vi "Identify Action.vi"(8 "error in (no error)":errorcluster, 10 "Item Tag":string) -> (0 "error out":errorcluster, 3 "RCM_Actions out":refnum<class "RCM_Actions.lvclass">)   [LabVIEW 2016, in "Assert API Components.lvlib" / "Assert Display.lvlib" / "Main Display.lvlib" / "RCM_Actions.lvclass"]
uses:
  RCM_Actions.lvclass
  Change Column Header/Change Column Header.lvclass
  D:/Work/Projects/actor_assert_api/Main Display/Right Click Menu Actions/RCM_Actions.lvclass
  Change Column Header/Change Column Header.lvclass/Change Column Header.ctl
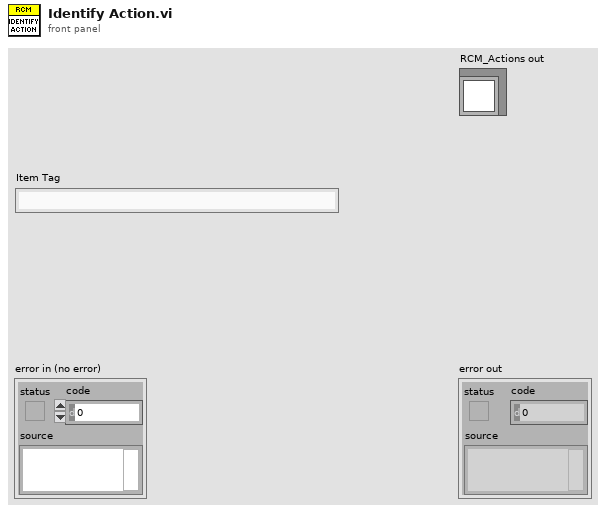
[diagram p1: front panel]
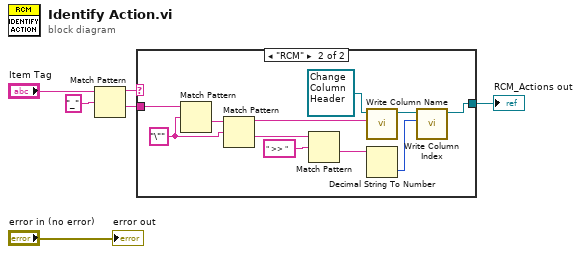
[diagram p0: block diagram]
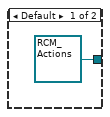
[diagram p2: hidden frame]
diagram:
  n1 = Match Pattern(string="Item Tag", regular expression="_") -> (before substring=w3:string, after substring=w4:string)  [unwired: 1 in, 2 out]
  n2 = case shown="\"RCM\"" w3 {
    tunnel: w4 -> [_ w13]
    tunnel: [refnum<class "RCM_Actions.lvclass"> refnum ("RCM_Actions out") w10] -> w2
    frame Default {
    }
    frame "RCM" {
      w17 = "\"" ("regular expression")
      n3 = Match Pattern(string=w13, regular expression=w17) -> (after substring=w18:string)  [unwired: 1 in, 3 out]
      n4 = Match Pattern(string=w18, regular expression=w17) -> (before substring=w9:string, after substring=w16:string)  [unwired: 1 in, 2 out]
      n5 = Match Pattern(string=w16, regular expression=" >> ") -> (after substring=w14:string)  [unwired: 1 in, 3 out]
      n6 = call "Write Column Name.vi"("Column Name"=w9, "Change Column Header in"=refnum<class "Change Column Header.lvclass"> refnum ("Assert API Components.lvlib:Assert Display.lvlib:Main Display.lvlib:Change Column Header.lvclass")) -> ("Change Column Header out"=w11:refnum<class "Change Column Header.lvclass">)  [unwired: 9 in]
      n7 = Decimal String To Number(string=w14) -> (number=w8:i32)  [unwired: 2 in, 1 out]
      n8 = call "Write Column Index.vi"("Column Index"=w8, "Change Column Header in"=w11) -> ("Change Column Header out"=w10:refnum<class "Change Column Header.lvclass">)  [unwired: 9 in]
    }
  }
  "RCM_Actions out" <- w2
  "error out" <- "error in (no error)"
